vi "Write Snake.vi"(8 "error in (no error)":errorcluster, 10 "Snake":refnum<class "Snake.lvclass">, 11 "Board Game in":refnum<class "Board Game.lvclass">) -> (0 "error out":errorcluster, 3 "Board Game out":refnum<class "Board Game.lvclass">)   [LabVIEW 2021, in "Board Game.lvclass"]
uses:
  Board Game.lvclass
  Snake_class/Snake.lvclass
  Board Game.lvclass/Board Game.ctl
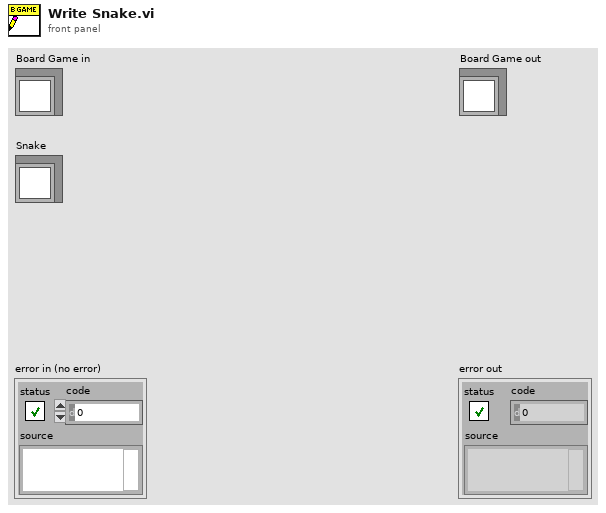
[diagram p1: front panel]
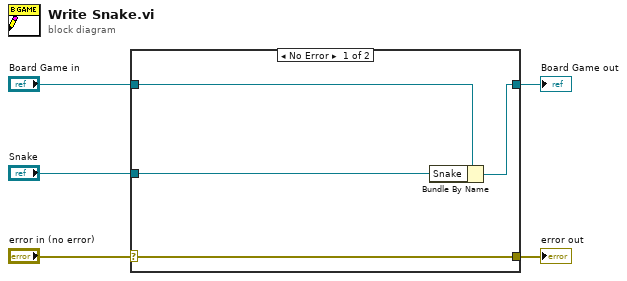
[diagram p0: block diagram]
diagram:
  n1 = case shown="No Error" "error in (no error)" {
    selector: "error in (no error)" -> [w9 w10]
    tunnel: [w9 w10] -> w4
    tunnel: [w7 w11] -> w2
    tunnel: "Board Game in" -> [w8 w11]
    tunnel: "Snake" -> [w6 _]
    frame No Error {
      n2 = Bundle By Name(cluster=w8, "Snake"=w6) -> (w7:refnum<class "Board Game.lvclass">)
    }
    frame Error {
    }
  }
  "error out" <- w4
  "Board Game out" <- w2
